vi "Get Value for cif_manager_OrchestrationLanguage_Flat.vi"(8 "error in (no error)":errorcluster, 10 "labview enum value":u32, 11 "gRPC ID":T1) -> (0 "error out":errorcluster, 2 "proto enum value":i32, 3 "gRPC ID Out":T1)   [LabVIEW 2021, in "CIF_Manager_client.lvlib"]
uses:
  CIF_Manager_client.lvlib
  <vilib>/gRPC/LabVIEW gRPC Library/Shared/grpcId.ctl
  <vilib>/gRPC/LabVIEW gRPC Library/Shared/TranslateGrpcError.vi
  <vilib>/gRPC/LabVIEW gRPC Library/Server API/Server/Get Server DLL Path.vi
  <vilib>/Utility/error.llb/Error Cluster From Error Code.vi
  <vilib>/gRPC/LabVIEW gRPC Library/grpc-lvsupport-release.lvlib
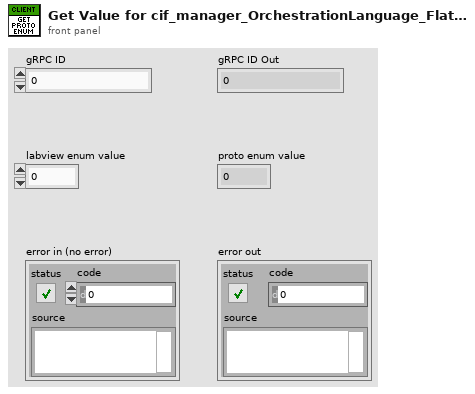
[diagram p1: front panel]
types:
  T1 = typedef "grpc-lvsupport-release.lvlib/grpcId.ctl" = u64
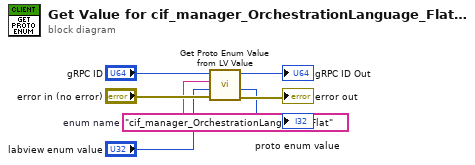
[diagram p0: block diagram]
diagram:
  w3 = "cif_manager_OrchestrationLanguage_Flat"  # enum name
  n1 = call <vilib>:"Get Proto Enum Value from LV Value.vi"("error in"="error in (no error)", "labview enum value"="labview enum value", "enum name"=w3, "gRPCid in"="gRPC ID") -> ("error out"=→"error out":errorcluster, "proto enum value"=→"proto enum value":i32, "gRPCid out"=→"gRPC ID Out":T1)  [unwired: 5 in]
